vi "Get Data.vi"(8 "error in (no error)":errorcluster, 10 "通道号":i32, 11 "VISA resource name":refnum<visa-resource-name>) -> (0 "error out":errorcluster, 2 "读取缓冲区":string, 3 "VISA resource name out":refnum<visa-resource-name>)   [LabVIEW 2015]
panel:
  in  "读取前延时(ms)":u32=500
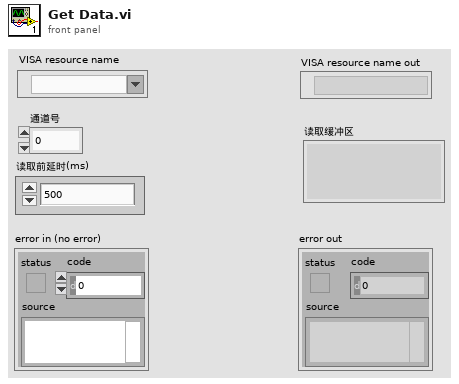
[diagram p1: front panel]
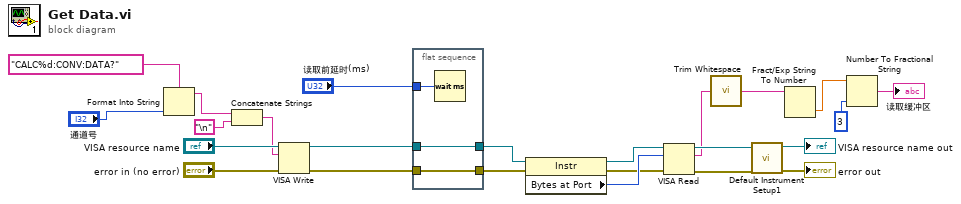
[diagram p0: block diagram]
diagram:
  n1 = Format Into String(format string="CALC%d:CONV:DATA?" ("Reset Command"), "通道号") -> (resulting string=w17:string)  [unwired: 2 in, 1 out]
  n2 = Concatenate Strings(w17, "\n") -> (w20:string)
  n3 = VISA Write(VISA resource name="VISA resource name", write buffer=w20, error in (no error)="error in (no error)") -> (VISA resource name out=w12:refnum<visa-resource-name>, error out=w11:errorcluster)  [unwired: 1 out]
  n4 = flat-sequence {
    tunnel: w11 -> [w26]
    tunnel: [w26] -> w9
    tunnel: w12 -> [w25]
    tunnel: [w25] -> w10
    tunnel: "读取前延时(ms)" -> [w27]
    frame #0 {
      n5 = Wait (ms)(milliseconds to wait=w27) -> ()  [unwired: 1 out]
    }
  }
  n6 = property class="Instr"(reference=w10, error in=w9) -> (reference out=w7:refnum<visa-resource-name>, error out=w6:errorcluster, "Bytes at Port"=w8:u32)
  n7 = VISA Read(VISA resource name=w7, byte count=w8, error in (no error)=w6) -> (VISA resource name out=w16:refnum<visa-resource-name>, read buffer=w5:string, error out=w15:errorcluster)  [unwired: 1 out]
  n8 = call <vilib>:"Trim Whitespace.vi"("string"=w5) -> ("trimmed string"=w4:string)  [unwired: 1 in]
  n9 = call "Default Instrument Setup1.vi"("error in (no error)"=w15, "VISA resource name"=w16) -> ("error out"=→"error out":errorcluster, "VISA resource name out"=→"VISA resource name out":refnum<visa-resource-name>)  [unwired: 8 in]
  n10 = Fract/Exp String To Number(string=w4) -> (number=w3:dbl)  [unwired: 3 in, 1 out]
  n11 = Number To Fractional String(number=w3, precision (6)=i16 3 ("精度(6)")) -> (F-format string=→"读取缓冲区":string)  [unwired: 2 in]
